vi "Main Monitor Loop.vi"(8 "error in (no error)":errorcluster, 11 "main ref":T1) -> (0 "error out":errorcluster)   [LabVIEW 2025]
uses:
  controls/LAB-IQ UI Data.ctl
panel:
  in  "millisecond multiple":u32=5
  out "Test Stop Temp":bool
  out "DepthZ":dbl
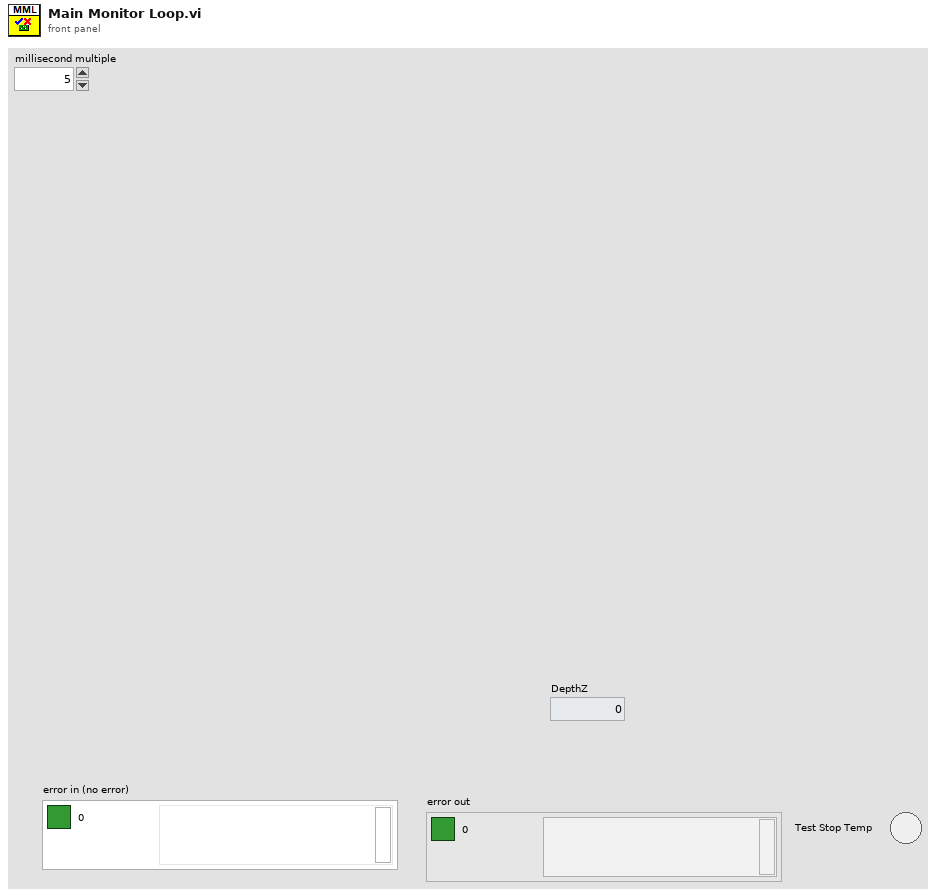
[diagram p1: front panel]
types:
  T1 = typedef "LAB-IQ UI Data.ctl" = cluster{"Main Home Screen":cluster{"GUI":refnum<vi>, "Platform Settings":refnum<vi>, "Configure":refnum<vi>, "Home":refnum<vi>, "EXIT":refnum<vi>, "service 2":refnum<vi>, "MainPage":refnum<vi>, "Analysis":refnum<vi>}, "Platform Settings":cluster{"mm/s  Surge":refnum<vi>, "Update Surge Speed":refnum<vi>, "Drive Error":refnum<vi>, "Disable Axis Jog Soft Limits":refnum<vi>, "mm/s  Sway":refnum<vi>, "Sway and Surge COM Status":refnum<vi>, "Heave COM Status":refnum<vi>, "Enable Platform":refnum<vi>, "Surge Forward Main":refnum<vi>, "Sway Right Main":refnum<vi>, "Sway Left Main":refnum<vi>, "Heave Down Main":refnum<vi>, "Heave Up main":refnum<vi>, "Update Sway Speed":refnum<vi>, "Update Heave Speed":refnum<vi>, "mm/s Heave":refnum<vi>, "mm/sec":refnum<vi>, "mm":refnum<vi>, "Surge Backward Main":refnum<vi>}, "Analysis Screen":cluster{"Analysis Home":refnum<vi>, "Surface Analysis":refnum<vi>, "Imaging":refnum<vi>, "Image Analysis":refnum<vi>, "Post Analysis":refnum<vi>}, "Config Screen":cluster{"Select Load Head":refnum<vi>, "Notes :":refnum<vi>, "FILE":refnum<vi>, "Sample ID :":refnum<vi>, "Operator ID :":refnum<vi>, "Operator Name :":refnum<vi>, "Auto":refnum<vi>}, "Motion Module":cluster{"zNL":refnum<vi>, "NL disp":refnum<vi>, "Rotary Tab":refnum<vi>, "Motion Direction:  3":refnum<vi>, "E.Velocity 2":refnum<vi>, "e.v/ssr 2":refnum<vi>, "Enter Fixed E.Velocity 2":refnum<vi>, "Enter Final SRR 2":refnum<vi>, "Enter initial SRR 2":refnum<vi>, "Enter Fixed SRR 2":refnum<vi>, "Enter the Final E.Velocity (m/s) 2":refnum<vi>, "Enter initial E.Velocity (m/s) 2":refnum<vi>, "Final Speed (RPM) 3":refnum<vi>, "Initial Speed (RPM) 2":refnum<vi>, "Enter the Final Velocity (m/s) 3":refnum<vi>, "Enter initial Velocity (m/s)  3":refnum<vi>, "Ramp Up 2":refnum<vi>, "TEST SELECTION":refnum<vi>, "SPEED SELECTION : ":refnum<vi>, "Angular Oscillation Set":refnum<vi>, "Traction":refnum<vi>, "Step Speed":refnum<vi>, "StepTable For Load-Speed":refnum<vi>, "StepTable For Speed":refnum<vi>, "Surge Forward MM":refnum<vi>, "Surge Backward MM":refnum<vi>, "M3 Image":refnum<vi>, "String 39":refnum<vi>, "Sway Left MM":refnum<vi>, "Sway Right MM":refnum<vi>, "Disable Axis Jog Soft Limits":refnum<vi>, "mm":refnum<vi>, "Heave Down MM":refnum<vi>, "Heave Up MM":refnum<vi>, "Wear Track Diameter (mm)":refnum<vi>, "Set WTD":refnum<vi>, "HomeScratch":refnum<vi>, "HomeRot":refnum<vi>, "PlaceModule":refnum<vi>, "Enter the Angle (Deg)":refnum<vi>, "Enter the Frequency (Hz)":refnum<vi>, "Motion Mode:":refnum<vi>, "LR Sway":refnum<vi>, "Rot Hor":refnum<vi>, "Scratch":refnum<vi>, "LR Cam":refnum<vi>, "MMBack":refnum<vi>, "MMNext":refnum<vi>, "Rot Ver":refnum<vi>, "Rotary Module Selection":refnum<vi>, "calculate rotary":refnum<vi>, "SPEED SELECTION : rotary":refnum<vi>, "Import 2":refnum<vi>, "Save 2":refnum<vi>, "File Path :  2":refnum<vi>, "String 45":refnum<vi>, "StepTable For Speed 3":refnum<vi>, "Enter the Speed(mm/sec)":refnum<vi>, "Enter the Speed(RPM)":refnum<vi>, "Enter Scratch Speed (mm/s):":refnum<vi>, "SwaySpeed Set":refnum<vi>, "Scartch Offset":refnum<vi>, "Motion type:":refnum<vi>, "HomeScratch 2":refnum<vi>, "Enter Scratch length (mm):":refnum<vi>, "Wear Track Diameter":refnum<vi>, "Rotary Speed Exced":refnum<vi>, "Scratch Mode":refnum<vi>, "No of Scratch":refnum<vi>}, "Environmental control":cluster{"Humidity  Status  3":refnum<vi>, "Low Temp  Status  2":refnum<vi>, "TK4 status 2":refnum<vi>, "Stage Temperature":refnum<vi>, "Sample Temperature":refnum<vi>, "Humidity (Amb)":refnum<vi>, "Clear List":refnum<vi>, "Add to list":refnum<vi>, "Wear":refnum<vi>, "Vibration":refnum<vi>, "Humidity (Chamber)":refnum<vi>, "Temperature (Chamber)":refnum<vi>, "ECR ":refnum<vi>, "Temperature (Amb)":refnum<vi>, "Microphone":refnum<vi>, "Acoustic Emission 3":refnum<vi>, "SNext":refnum<vi>, "APBack":refnum<vi>, "Enter the Temperature (°C):":refnum<vi>, "Enter the Stage \nTemperature (°C):":refnum<vi>, "Enter the Humidity (%Rh):":refnum<vi>, "Low Temp":refnum<vi>, "High Temp":refnum<vi>, "Humidity":refnum<vi>, "Sensors Picked":refnum<vi>}, "About Screen":cluster{"Password":refnum<vi>, "Home Service":refnum<vi>, "Advanced Setting":refnum<vi>, "About Tab":refnum<vi>, "ECR Port:":refnum<vi>, "Ramp Port:":refnum<vi>, "Installation/Replacement completed":refnum<vi>, "Loahead":refnum<vi>, "Heave and Surge COM Port:":refnum<vi>, "Sway COM Port:":refnum<vi>, "Temp Modbus:":refnum<vi>, "Humidity Port:":refnum<vi>, "Edit Gain Constants":refnum<vi>, "Save Gain Constants":refnum<vi>}, "Main Screen":cluster{"Main Screen Tab":refnum<vi>, "Angle and Frequency":refnum<vi>, "Stroke (mm)":refnum<vi>, "Angle (Deg)":refnum<vi>, "Main Speed Tab":refnum<vi>, "MTM MOTOR DISPLAY":refnum<vi>, "Disc Speed (m/sec)":refnum<vi>, "Ball Speed (m/sec)":refnum<vi>, "Disc Speed (RPM)":refnum<vi>, "Ball Speed (RPM)":refnum<vi>, "SPEED TAB":refnum<vi>, "Speed (m/sec)":refnum<vi>, "Set Speed (m/sec)":refnum<vi>, "Speed (RPM)":refnum<vi>, "Set Speed":refnum<vi>, "Time Tab":refnum<vi>, "Time ( HH:MM:SS ) 2":refnum<vi>, "Test Duration":refnum<vi>, "Test Duration 4":refnum<vi>, "TEST CYCLE":refnum<vi>, "TOTAL CYCLES":refnum<vi>, "Set Load (N)":refnum<vi>, "Temp Tabs":refnum<vi>, "Heater":refnum<vi>, "TK4 status":refnum<vi>, "ChamberTemp":refnum<vi>, "SetTmp":refnum<vi>, "Controller  Status":refnum<vi>, "ChamberTemp 2":refnum<vi>, "SetTmp 2":refnum<vi>, "Controller  Status 2":refnum<vi>, "ChamberTemp 3":refnum<vi>, "SetTmp 3":refnum<vi>, "Cooling":refnum<vi>, "Load Communication":refnum<vi>, "Ambient \nTemperature":refnum<vi>, "HumCOMStatus":refnum<vi>, "Ambient\n Humidity":refnum<vi>, "Freq (Hz)":refnum<vi>, "Load En":refnum<vi>, "NLt":refnum<vi>, "zNL 2":refnum<vi>, "Humidity On":refnum<vi>, "humidity disp":refnum<vi>, "Set Humidity":refnum<vi>, "NL disp 2":refnum<vi>, "Humidity On 2":refnum<vi>, "humidity disp 2":refnum<vi>, "Set Humidity 2":refnum<vi>, "NL disp 3":refnum<vi>, "AppLoadSeq scratch":refnum<vi>, "Stop Scratch":refnum<vi>, "ClrLog":refnum<vi>, "Trip Log":refnum<vi>, "STOP":refnum<vi>, "Start Test":refnum<vi>, "Test status":refnum<vi>, "AR Led":refnum<vi>, "Data":refnum<vi>, "Health":refnum<vi>, "Sway COM Status":refnum<vi>, "Heave COM Status":refnum<vi>, "Grp Tab":refnum<vi>, "Sub Graph":refnum<vi>, "SD (mm)":refnum<vi>, "Siliding distance Reset Graph":refnum<vi>, "SDGp":refnum<vi>, "Humidity Reset Graph":refnum<vi>, "HumrGp":refnum<vi>, "Acoustic Emission (mV)":refnum<vi>, "Aqucostic Reset Graph":refnum<vi>, "gACQUOS":refnum<vi>, "ECR RESET":refnum<vi>, "ECR":refnum<vi>, "Temperature Reset":refnum<vi>, "Acoustic Emission (mV) 2":refnum<vi>, "Aqucostic Reset Graph 2":refnum<vi>, "gACQUOS 2":refnum<vi>, "ECR RESET 2":refnum<vi>, "ECR 2":refnum<vi>, "Temperature Reset 2":refnum<vi>, "Temperature (deg c)":refnum<vi>, "Speed Reset Graph":refnum<vi>, "Speed Tab":refnum<vi>, "MTM DISC  SPEED":refnum<vi>, "MTM BALL SPEED":refnum<vi>, "speed mm/sec":refnum<vi>, "Hymidity":refnum<vi>, "Humidity Disable trip":refnum<vi>, "CoF Trip  2":refnum<vi>, "Depth Trip":refnum<vi>, "Weart Deapth":refnum<vi>, "Depth Reset Graph":refnum<vi>, "Weart":refnum<vi>, "Depthz":refnum<vi>, "Depth (µm)":refnum<vi>, "WearGp":refnum<vi>, "NL Trip 2":refnum<vi>, "Load pid":refnum<vi>, "Load Disable Trip":refnum<vi>, "Load Reset Graph":refnum<vi>, "NL Display 4":refnum<vi>, "Main Chart 3":refnum<vi>, "BACK":refnum<vi>, "Depth Trip 2":refnum<vi>, "COF TRIP ":refnum<vi>, "Friction Force (N)":refnum<vi>, "FF Reset Graph":refnum<vi>, "FF Disable Trip":refnum<vi>, "FF TRIP":refnum<vi>, "COF Disable Trip":refnum<vi>, "COF Reset Graph":refnum<vi>, "Start Test Temp":refnum<vi>, "zFF":refnum<vi>, "Friction Force (N) Graph":refnum<vi>, "Coefficient of Friction":refnum<vi>, "Scratch Start Test":refnum<vi>, "FF Tab":refnum<vi>, "Cyclic Friction Force (N)":refnum<vi>, "CZ FF":refnum<vi>, "Cyclic Friction Force (N) Graph":refnum<vi>, "Cyclic Coefficient of Friction":refnum<vi>, "Cyclic FF TRIP":refnum<vi>, "Cyclic FF Disable Trip":refnum<vi>, "cyclic COF Disable Trip":refnum<vi>, "cyclic COF TRIP":refnum<vi>, "cyclic COF Reset Graph":refnum<vi>, "Cyclic FF Reset Graph":refnum<vi>, "Test Trip":refnum<vi>, "Multi Scratch Pass":refnum<vi>}, "Loading":cluster{"Indentation":refnum<vi>, "Reference Sample":refnum<vi>, "Load Cell Communication Slide":refnum<vi>, "com 3":refnum<vi>, "com":refnum<vi>, "DecaForce COM Status":refnum<vi>, "Update":refnum<vi>, "Clear 3":refnum<vi>, "seq":refnum<vi>, "Stribeck table":refnum<vi>, "Stribeck Table  For loading":refnum<vi>, "Loading Mode":refnum<vi>, "Enter the Final Load (N)":refnum<vi>, "Enter the CoF Trip":refnum<vi>, "Enter the Friction Force Trip":refnum<vi>, "Enter the Normal load Trip":refnum<vi>, "Enter the Load  (N)":refnum<vi>, "KiloForce":refnum<vi>, "DecaForce ":refnum<vi>, "MicroForce":refnum<vi>, "LHBack":refnum<vi>, "LHNext":refnum<vi>, "Enter the Loading Rate (N/min)":refnum<vi>, "Message":refnum<vi>, "Warning 2":refnum<vi>, "SSP 0.75":refnum<vi>, "SSP 0.5":refnum<vi>, "SSP 0.3":refnum<vi>, "Warning":refnum<vi>, "gui GIF":refnum<vi>, "Communication is established":refnum<vi>, "AppLoad 4":refnum<vi>, "Multipoint":refnum<vi>, "Load Selection":refnum<vi>}, "PID":cluster{"Ramp MulFac":refnum<vi>, "pulses LoadDiffRamp(2..10)":refnum<vi>, "PulseControlRamp(diff<=3N)":refnum<vi>, "SetLoadDeadband(%) Load(0-10N)":refnum<vi>, "PID gains out delay (microForce)":refnum<vi>, "Ramp":refnum<vi>, "Gain 2":refnum<vi>, "pulses LoadDiff(2..10)":refnum<vi>, "pulses LoadDiff(11..50)":refnum<vi>, "PulseControl(diff<=3N)":refnum<vi>, "SetLoadDeadband(%)  2":refnum<vi>, "Dummy Run":refnum<vi>, "Vertical load (N)":refnum<vi>, "AutoTune":refnum<vi>, "Offset 3 ":refnum<vi>, "apply load":refnum<vi>, "Offset  3":refnum<vi>, "apply load 2":refnum<vi>, "Enter ByPass Load":refnum<vi>, "reinit 3":refnum<vi>, "output range delay":refnum<vi>, "PID gains out delay":refnum<vi>, "Bypass Load":refnum<vi>, "pulsesSent":refnum<vi>, "pulses ":refnum<vi>, "actpid":refnum<vi>, "gFF Rot":refnum<vi>, "pulses LoadDiff(21..1000)":refnum<vi>, "Delay":refnum<vi>, "deadband":refnum<vi>}, "Config Parameters":cluster{"Tab Control 3":refnum<vi>, "Tab Control 19":refnum<vi>, "SAMPLES":refnum<vi>, "Re-initilaize":refnum<vi>, "Filter ON/OFF":refnum<vi>, "TracHomeSurgeOffsetCounts 10MM":refnum<vi>, "TracHomeSwayOffsetCounts 10MM":refnum<vi>, "Acoustic Emission:":refnum<vi>, "Apply Filter (FF)":refnum<vi>, "Filter% 2":refnum<vi>, "Apply Filter (Load)":refnum<vi>, "Filter% ":refnum<vi>, "Sway distance (mm)":refnum<vi>, "Surge distance (mm)":refnum<vi>, "DataSavingLoopDelay(ms)":refnum<vi>, "SAVE 2":refnum<vi>, "Enter Distance":refnum<vi>, "Sway Counts:":refnum<vi>, "Distance (mm): 3":refnum<vi>, "Surge Counts:":refnum<vi>, "Distance (mm): 2":refnum<vi>, "Distance (mm):":refnum<vi>, "Heave Counts:":refnum<vi>, "LRMHomeSurgeOffsetCounts":refnum<vi>, "LRMHomeSwayOffsetCounts":refnum<vi>, "TracHomeSurgeOffsetCounts 20MM":refnum<vi>, "TracHomeSwayOffsetCounts 20MM":refnum<vi>, "RotHomeSwayOffsetCounts":refnum<vi>, "RotHomeSurgeOffsetCounts":refnum<vi>, "Heave distance":refnum<vi>, "Zmm":refnum<vi>, "Heave Pulses/mm":refnum<vi>, "Surge Pulses/mm":refnum<vi>, "Sway Pulses/mm":refnum<vi>, "Heave Pitch":refnum<vi>, "Surge Pitch":refnum<vi>, "Sway Pitch":refnum<vi>, "Heave PPR":refnum<vi>, "Surge PPR":refnum<vi>, "Sway PPR":refnum<vi>, "Tab Control 5":refnum<vi>, "Tab Control 14":refnum<vi>, "Tab Control 26":refnum<vi>, "AE":refnum<vi>, "Heave Loop Delay":refnum<vi>, "Heave PID Speed":refnum<vi>, "Surge Jog Speed":refnum<vi>, "Heave Jog Speed":refnum<vi>, "Sway Loop Delay":refnum<vi>, "Sway PID Speed":refnum<vi>, "Sway Jog Speed":refnum<vi>}, "Loading Com Port":cluster{"ClearAll":refnum<vi>, "Mz(Nm)":refnum<vi>, "My(Nm)":refnum<vi>, "Mx(Nm)":refnum<vi>, "Save Dwell":refnum<vi>, "Mx ":refnum<vi>, "My ":refnum<vi>, "Mz":refnum<vi>, "Fx(N)":refnum<vi>, "Fy(N)":refnum<vi>, "Fz(N)":refnum<vi>, "ZeroAll":refnum<vi>, "Acq Delay (ms)":refnum<vi>, "Burst Delay (ms)":refnum<vi>, "model":refnum<vi>, "SN":refnum<vi>, "FFx(N)":refnum<vi>, "Sensor IP":refnum<vi>, "Port":refnum<vi>, "FFy(N)":refnum<vi>, "Load(N)":refnum<vi>, "delete Handle":refnum<vi>, "Create Handle":refnum<vi>, "ft_data":refnum<vi>, "ft_range":refnum<vi>, "ft_data 2":refnum<vi>, "stop 6":refnum<vi>, "running_flag":refnum<vi>, "ft_udp_handle":refnum<vi>, "get-data-return":refnum<vi>, "get-range-return":refnum<vi>, "zero-return":refnum<vi>, "filter-return":refnum<vi>, "initial-return":refnum<vi>, "deleteHandle-result":refnum<vi>, "Load Cell Temp":refnum<vi>}, "Heave AND Surge":cluster{"SURGE POSE":refnum<vi>, "error out Read":refnum<vi>, "HEAVE POSE":refnum<vi>, "State":refnum<vi>, "Homed":refnum<vi>, "Sequence ID":refnum<vi>, "error out Write":refnum<vi>, "faultCode":refnum<vi>, "Ack ID":refnum<vi>, "SPEED":refnum<vi>, "Distance":refnum<vi>, "Mode Command":refnum<vi>, "Heave and Surge Read":refnum<vi>, "Read Heave Temp":refnum<vi>, "Spare 15":refnum<vi>, "Spare 14":refnum<vi>, "Spare 13":refnum<vi>, "Spare 12":refnum<vi>, "Spare 11":refnum<vi>, "Spare 10":refnum<vi>, "Spare 9":refnum<vi>, "Spare 8":refnum<vi>, "Spare 7":refnum<vi>, "Spare 6":refnum<vi>, "Spare 5":refnum<vi>, "Spare 4":refnum<vi>, "Spare 2":refnum<vi>, "Spare 1":refnum<vi>, "Node Id":refnum<vi>, "Spare 3":refnum<vi>, "SPARE 4":refnum<vi>, "SPARE 3":refnum<vi>, "SPARE 2":refnum<vi>, "SPARE 1":refnum<vi>, "fwMajor":refnum<vi>, "fwMinor":refnum<vi>, "Manual Write":refnum<vi>, "Heave and Surge Write":refnum<vi>}, "New PID LOGIC":cluster{"Fine Tune Zone":refnum<vi>, "PID SDelay":refnum<vi>, "Max_pos_limit":refnum<vi>, "Min_pos_limit":refnum<vi>, "i_limit":refnum<vi>, "pct_scale":refnum<vi>, "Deadband":refnum<vi>, "Kd":refnum<vi>, "Ki":refnum<vi>, "Kp":refnum<vi>, "Current Position":refnum<vi>, "Set Load":refnum<vi>, "Current Load":refnum<vi>, "Pulse delta":refnum<vi>, "Init Step":refnum<vi>, "Max Step Linit":refnum<vi>}, "SWAY ":cluster{"fwMajor":refnum<vi>, "Homed":refnum<vi>, "Rotary POSE":refnum<vi>, "State":refnum<vi>, "SWAY POSE":refnum<vi>, "Ack ID":refnum<vi>, "faultCode":refnum<vi>, "Node Id":refnum<vi>, "fwMinor":refnum<vi>, "Spare 6":refnum<vi>, "Spare 5":refnum<vi>, "Spare 4":refnum<vi>, "Spare 3":refnum<vi>, "Spare 2":refnum<vi>, "Spare 1":refnum<vi>, "Spare 7":refnum<vi>, "SPARE  5":refnum<vi>, "error out Write  SWAY ":refnum<vi>, "error out Read SWAY ":refnum<vi>, "Manual Write SWAY ":refnum<vi>, "SWAY WRITE":refnum<vi>, "SPARE  4":refnum<vi>, "SPARE  3":refnum<vi>, "SPARE 2":refnum<vi>, "SPARE 1":refnum<vi>, "Spare 15":refnum<vi>, "Spare 14":refnum<vi>, "Spare 13":refnum<vi>, "Spare 12":refnum<vi>, "Spare 11":refnum<vi>, "Spare 9":refnum<vi>, "Spare 8":refnum<vi>, "SPEED":refnum<vi>, "Distance":refnum<vi>, "Mode Command":refnum<vi>, "Sequence ID":refnum<vi>, "SWAY READ":refnum<vi>, "Spare 10":refnum<vi>, "Read SWAY Temp":refnum<vi>}, "Analysis Screen":cluster{"Analysis Home":refnum<vi>, "Refresh 2":refnum<vi>, "MEAN 4":refnum<vi>, "SD 4":refnum<vi>, "VARIANCE 4":refnum<vi>, "MEAN  3":refnum<vi>, "SD  3":refnum<vi>, "VARIANCE  3":refnum<vi>, "MEAN 2":refnum<vi>, "SD  2":refnum<vi>, "VARIANCE 2":refnum<vi>, "MEAN":refnum<vi>, "SD":refnum<vi>, "VARIANCE":refnum<vi>, "File 4 Discription":refnum<vi>, "OPEN 4":refnum<vi>, "File Name 4":refnum<vi>, "OPEN 3":refnum<vi>, "File 3 Discription":refnum<vi>, "File Name 3":refnum<vi>, "Y-AXIS":refnum<vi>, "X-AXIS":refnum<vi>, "XY Graph":refnum<vi>, "File Name 2":refnum<vi>, "File Name 1":refnum<vi>, "OPEN 2":refnum<vi>, "OPEN 1":refnum<vi>, "File 1 Discription ":refnum<vi>, "File 2 Discription":refnum<vi>}}
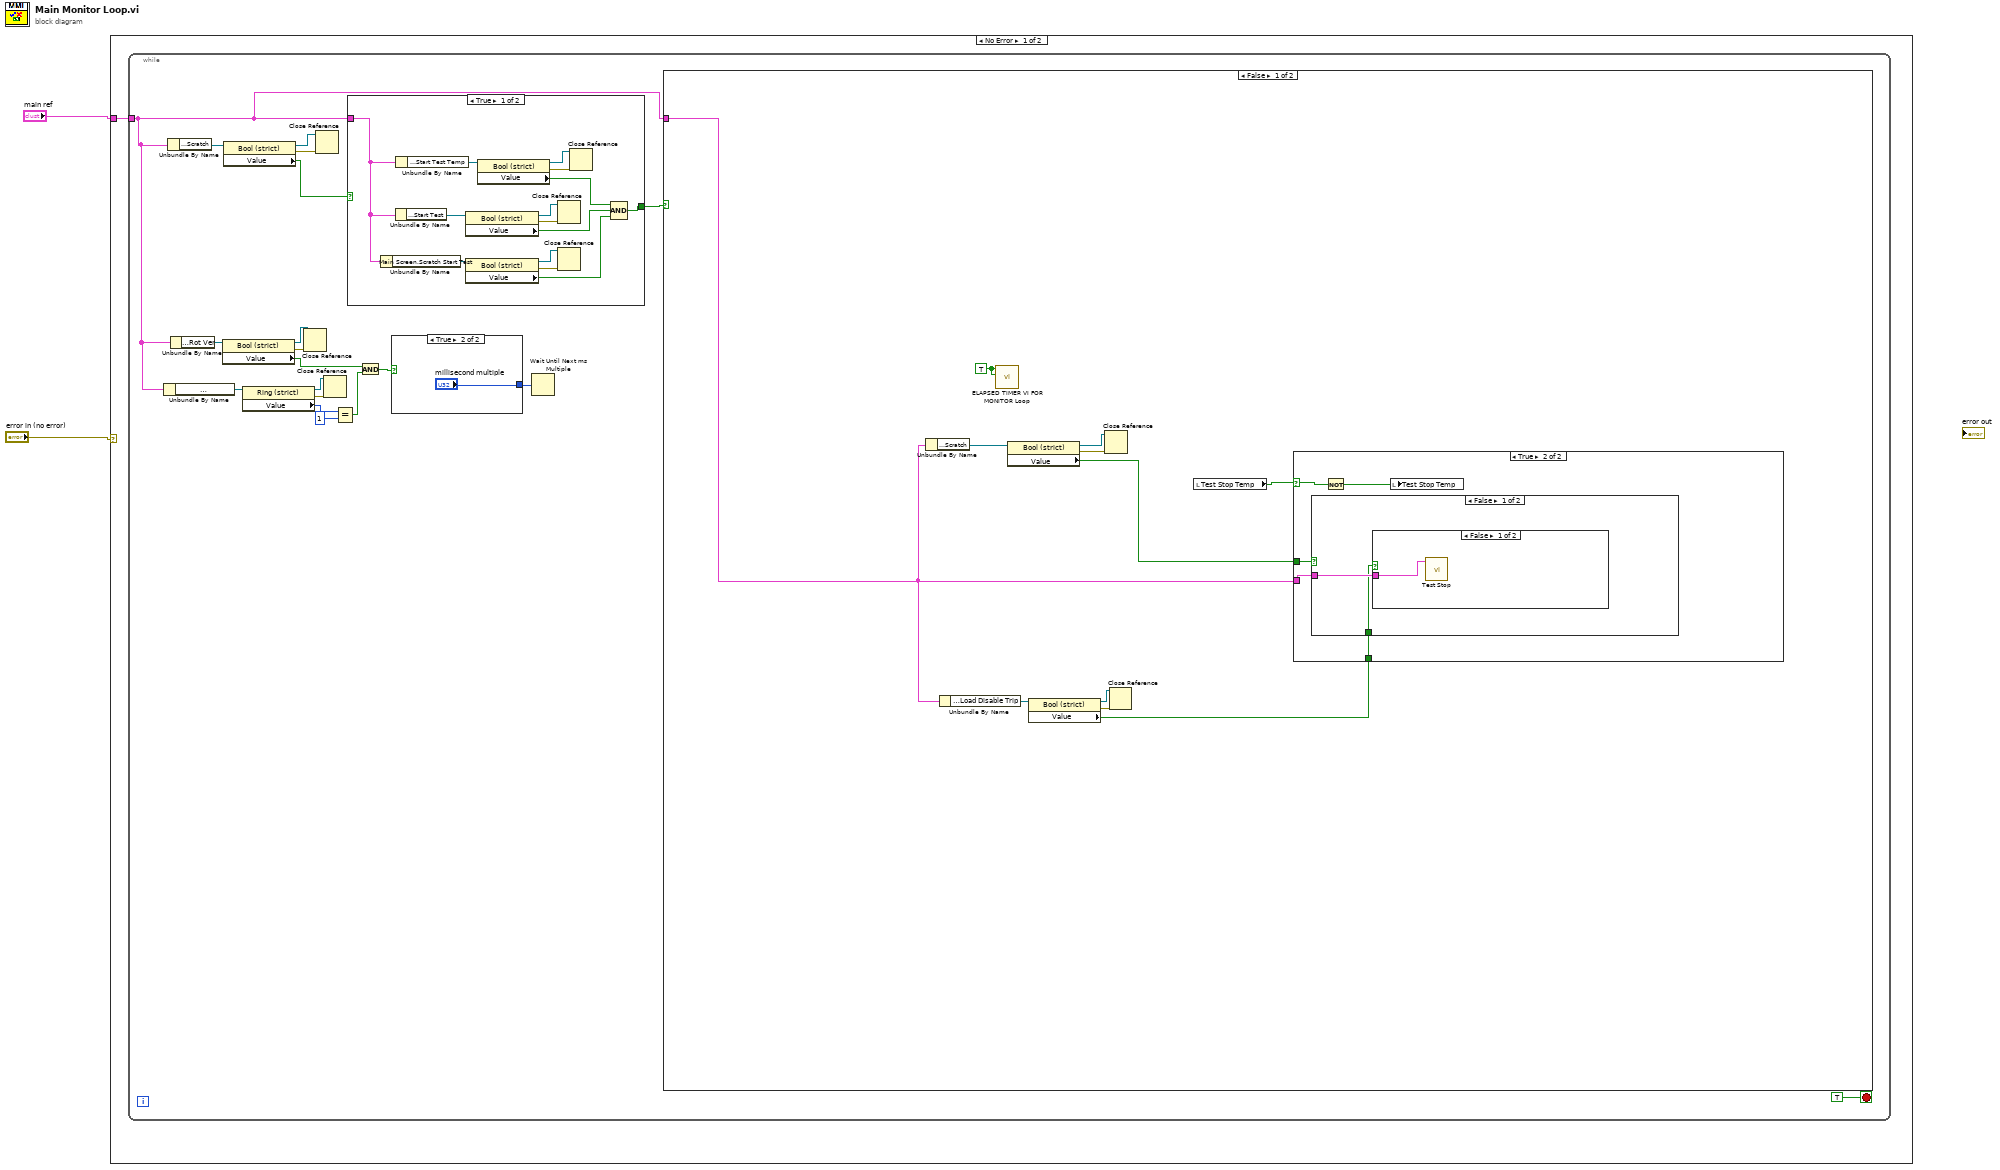
[diagram p0: block diagram]
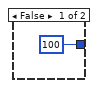
[diagram p2: hidden frame]
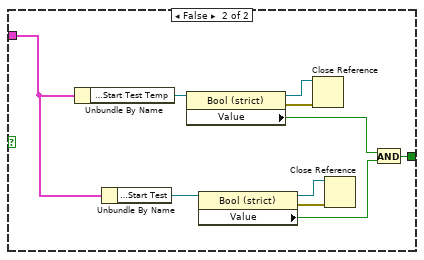
[diagram p3: hidden frame]
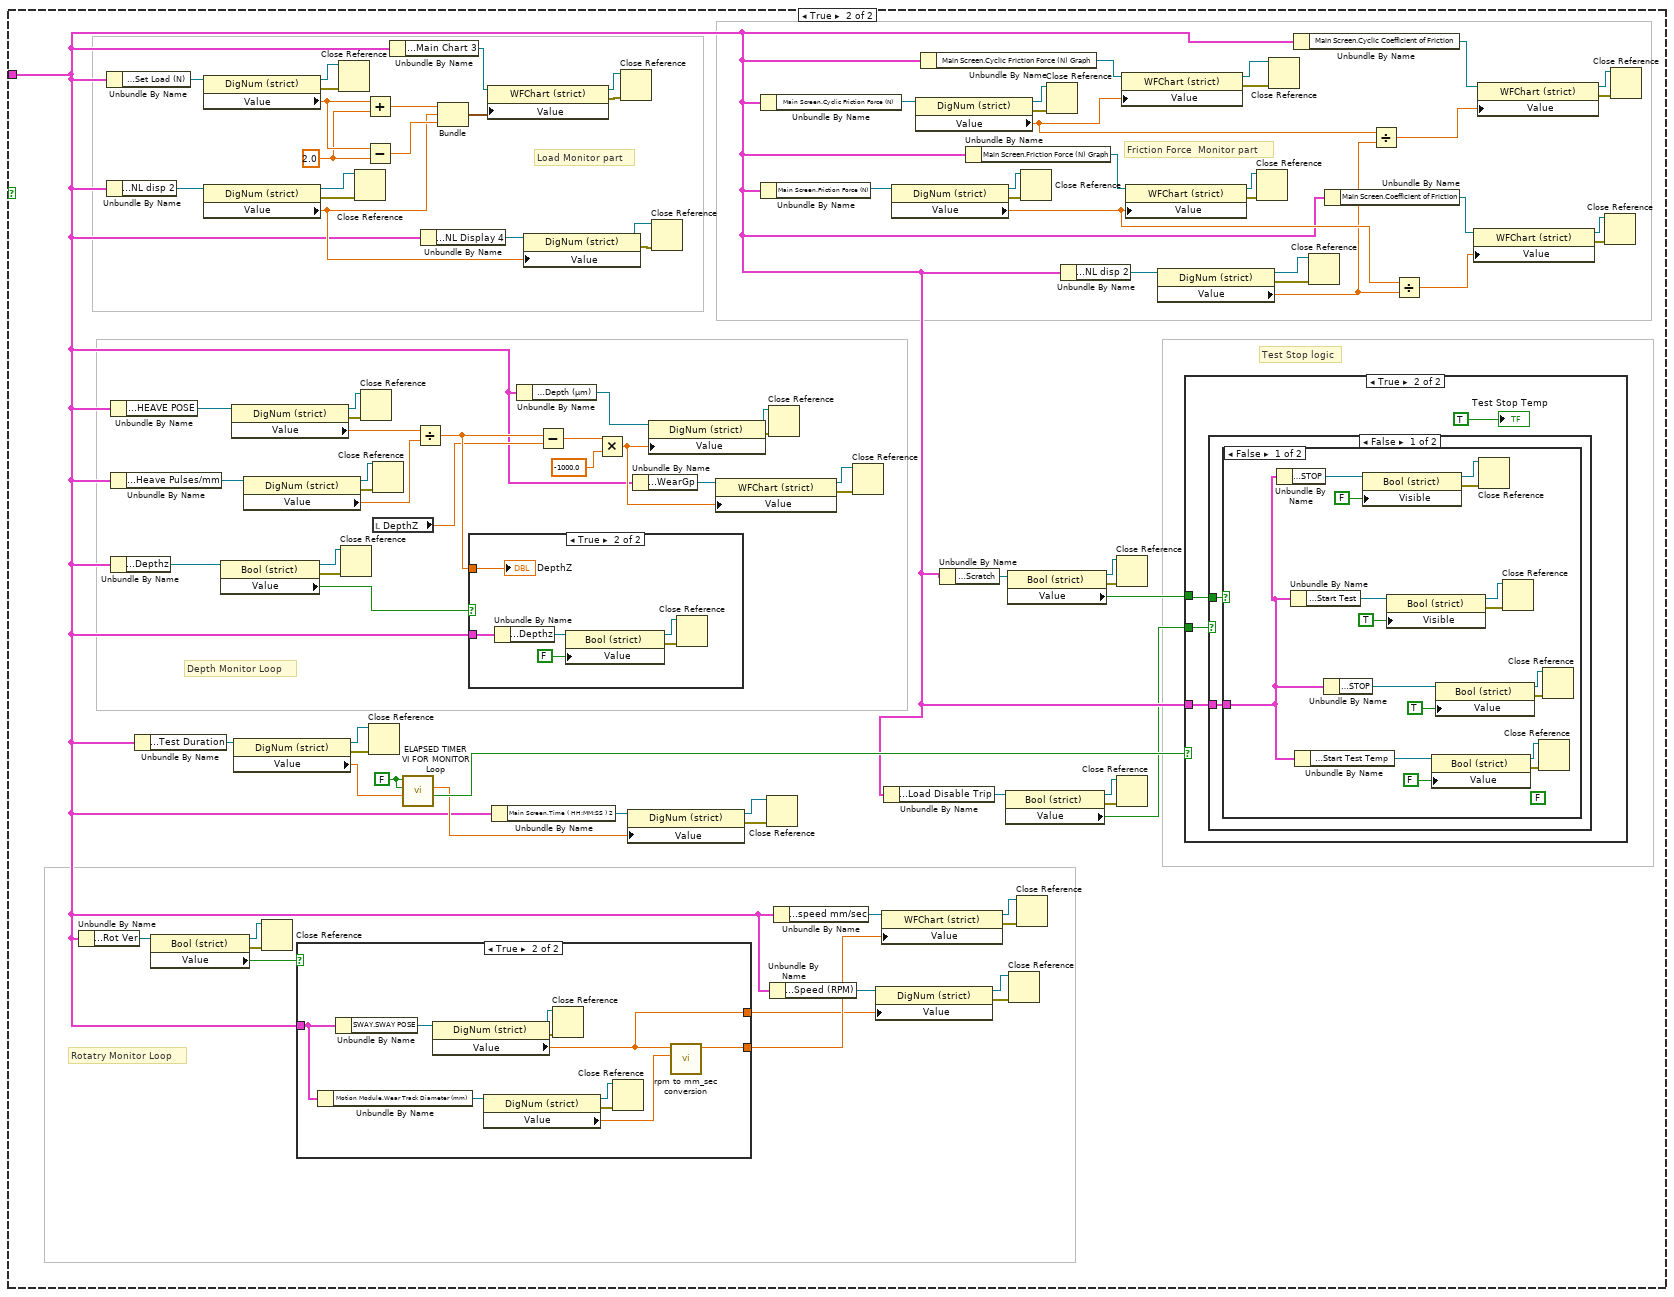
[diagram p7: hidden frame]
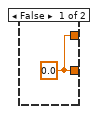
[diagram p8: hidden frame]
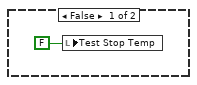
[diagram p9: hidden frame]
diagram:
  n1 = case shown="No Error" "error in (no error)" {
    tunnel: "main ref" -> [w3 _]
    frame No Error {
      n2 = while {
        tunnel: w3 -> [w5]
        stop <- TRUE stop-if-true
        n3 = Unbundle By Name(w5) -> ("Motion Module.Motion Mode:"=w10:refnum<vi>)
        n4 = Unbundle By Name(w5) -> ("Motion Module.Scratch"=w19:refnum<vi>)
        n5 = Unbundle By Name(w5) -> ("Motion Module.Rot Ver"=w15:refnum<vi>)
        n6 = property class="Bool (strict)"(reference=w15) -> (reference out=w13:refnum<vi>, error out=w14:errorcluster, "Value"=w7:bool)  [unwired: 1 in]
        n7 = property class="Bool (strict)"(reference=w19) -> (reference out=w20:refnum<vi>, error out=w18:errorcluster, "Value"=w17:bool)  [unwired: 1 in]
        n8 = property class="Ring (strict)"(reference=w10) -> (reference out=w12:refnum<vi>, error out=w11:errorcluster, "Value"=w9:u16)  [unwired: 1 in]
        n9 = Close Reference(reference=w13, error in (no error)=w14) -> ()  [unwired: 1 out]
        n10 = Close Reference(reference=w20, error in (no error)=w18) -> ()  [unwired: 1 out]
        n11 = Close Reference(reference=w12, error in (no error)=w11) -> ()  [unwired: 1 out]
        n12 = Equal?(x=w9, y=u16 1) -> (x = y?=w6:bool)
        n13 = case shown="True" w17 {
          tunnel: w5 -> [w26 w42]
          tunnel: [w30 w40] -> w21
          frame True {
            n14 = Unbundle By Name(w26) -> ("Main Screen.Scratch Start Test"=w28:refnum<vi>)
            n15 = Unbundle By Name(w26) -> ("Main Screen.Start Test"=w34:refnum<vi>)
            n16 = Unbundle By Name(w26) -> ("Main Screen.Start Test Temp"=w37:refnum<vi>)
            n17 = property class="Bool (strict)"(reference=w34) -> (reference out=w33:refnum<vi>, error out=w35:errorcluster, "Value"=w31:bool)  [unwired: 1 in]
            n18 = property class="Bool (strict)"(reference=w28) -> (reference out=w29:refnum<vi>, error out=w27:errorcluster, "Value"=w25:bool)  [unwired: 1 in]
            n19 = property class="Bool (strict)"(reference=w37) -> (reference out=w38:refnum<vi>, error out=w36:errorcluster, "Value"=w32:bool)  [unwired: 1 in]
            n20 = Close Reference(reference=w33, error in (no error)=w35) -> ()  [unwired: 1 out]
            n21 = Close Reference(reference=w29, error in (no error)=w27) -> ()  [unwired: 1 out]
            n22 = Close Reference(reference=w38, error in (no error)=w36) -> ()  [unwired: 1 out]
            n23 = Compound Arithmetic op=AND(w32, w31, w25) -> (w30:bool)
          }
          frame False {
            n24 = Unbundle By Name(w42) -> ("Main Screen.Start Test Temp"=w47:refnum<vi>)
            n25 = Unbundle By Name(w42) -> ("Main Screen.Start Test"=w44:refnum<vi>)
            n26 = property class="Bool (strict)"(reference=w47) -> (reference out=w48:refnum<vi>, error out=w46:errorcluster, "Value"=w41:bool)  [unwired: 1 in]
            n27 = property class="Bool (strict)"(reference=w44) -> (reference out=w43:refnum<vi>, error out=w45:errorcluster, "Value"=w39:bool)  [unwired: 1 in]
            n28 = Close Reference(reference=w48, error in (no error)=w46) -> ()  [unwired: 1 out]
            n29 = Close Reference(reference=w43, error in (no error)=w45) -> ()  [unwired: 1 out]
            n30 = And(x=w41, y=w39) -> (x .and. y?=w40:bool)
          }
        }
        n31 = And(x=w7, y=w6) -> (x .and. y?=w4:bool)
        n32 = case shown="True" w4 {
          tunnel: [u32 100 ("millisecond multiple") "millisecond multiple"] -> w16
          frame False {
          }
          frame True {
          }
        }
        n33 = Wait Until Next ms Multiple(millisecond multiple=w16) -> ()  [unwired: 1 out]
        n34 = case shown="False" w21 {
          tunnel: w5 -> [w50 w69]
          frame False {
            w59 = TRUE ("PAUSE")
            n35 = Unbundle By Name(w50) -> ("Motion Module.Scratch"=w57:refnum<vi>)
            n36 = Unbundle By Name(w50) -> ("Main Screen.Load Disable Trip"=w51:refnum<vi>)
            n37 = call "ELAPSED TIMER VI FOR MONITOR Loop.vi"("RESET"=w59, "PAUSE"=w59) -> ()  [unwired: 7 in, 3 out]
            n38 = property class="Bool (strict)"(reference=w57) -> (reference out=w55:refnum<vi>, error out=w56:errorcluster, "Value"=w54:bool)  [unwired: 1 in]
            n39 = property class="Bool (strict)"(reference=w51) -> (reference out=w53:refnum<vi>, error out=w52:errorcluster, "Value"=w49:bool)  [unwired: 1 in]
            n40 = Close Reference(reference=w55, error in (no error)=w56) -> ()  [unwired: 1 out]
            n41 = Close Reference(reference=w53, error in (no error)=w52) -> ()  [unwired: 1 out]
            n42 = local read "Test Stop Temp"() -> (w58:bool)
            n43 = case shown="True" w58 {
              selector: w58 -> [_ w64]
              tunnel: w50 -> [_ w62]
              tunnel: w54 -> [_ w61]
              tunnel: w49 -> [_ w60]
              frame False {
              }
              frame True {
                n44 = case shown="False" w61 {
                  tunnel: w62 -> [w66 _]
                  tunnel: w60 -> [w65 _]
                  frame False {
                    n45 = case shown="False" w65 {
                      tunnel: w66 -> [w67 _]
                      frame False {
                        n46 = call "Test Stop.vi"("Data Cluster"=w67) -> ()  [unwired: 10 in, 1 out]
                      }
                      frame True {
                      }
                    }
                  }
                  frame True {
                  }
                }
                n47 = Not(x=w64) -> (.not. x?=w63:bool)
                n48 = local write "Test Stop Temp"(w63) -> ()
              }
            }
          }
          frame True {
            w125 = FALSE ("PAUSE")
            w153 = 2.0 ("y")
            # "Rotatry Monitor Loop"
            # "Test Stop logic"
            # "Depth Monitor Loop"
            # "Friction Force  Monitor part"
            # "Load Monitor part"
            n49 = Unbundle By Name(w69) -> ("Motion Module.Rot Ver"=w84:refnum<vi>)
            n50 = Unbundle By Name(w69) -> ("Main Screen.Set Load (N)"=w155:refnum<vi>)
            n51 = Unbundle By Name(w69) -> ("Main Screen.NL disp 2"=w165:refnum<vi>)
            n52 = Unbundle By Name(w69) -> ("Heave AND Surge.HEAVE POSE"=w147:refnum<vi>)
            n53 = Unbundle By Name(w69) -> ("Config Parameters.Heave Pulses/mm"=w144:refnum<vi>)
            n54 = Unbundle By Name(w69) -> ("Main Screen.Depthz"=w139:refnum<vi>)
            n55 = Unbundle By Name(w69) -> ("Main Screen.Test Duration"=w123:refnum<vi>)
            n56 = property class="Bool (strict)"(reference=w84) -> (reference out=w82:refnum<vi>, error out=w83:errorcluster, "Value"=w81:bool)  [unwired: 1 in]
            n57 = property class="DigNum (strict)"(reference=w155) -> (reference out=w149:refnum<vi>, error out=w156:errorcluster, "Value"=w154:dbl)  [unwired: 1 in]
            n58 = property class="DigNum (strict)"(reference=w165) -> (reference out=w163:refnum<vi>, error out=w164:errorcluster, "Value"=w100:dbl)  [unwired: 1 in]
            n59 = property class="Bool (strict)"(reference=w139) -> (reference out=w140:refnum<vi>, error out=w138:errorcluster, "Value"=w137:bool)  [unwired: 1 in]
            n60 = property class="DigNum (strict)"(reference=w147) -> (reference out=w148:refnum<vi>, error out=w146:errorcluster, "Value"=w142:sgl)  [unwired: 1 in]
            n61 = property class="DigNum (strict)"(reference=w123) -> (reference out=w124:refnum<vi>, error out=w122:errorcluster, "Value"=w121:dbl)  [unwired: 1 in]
            n62 = property class="DigNum (strict)"(reference=w144) -> (reference out=w143:refnum<vi>, error out=w145:errorcluster, "Value"=w141:dbl)  [unwired: 1 in]
            n63 = Close Reference(reference=w82, error in (no error)=w83) -> ()  [unwired: 1 out]
            n64 = case shown="True" w81 {
              tunnel: w69 -> [_ w170]
              tunnel: [w166 w168] -> w77
              tunnel: [w166 w167] -> w73
              frame False {
                w166 = 0.0 ("Enter initial Velocity (m/s)  4")
              }
              frame True {
                n65 = Unbundle By Name(w170) -> ("Motion Module.Wear Track Diameter (mm)"=w173:refnum<vi>)
                n66 = Unbundle By Name(w170) -> ("SWAY.SWAY POSE"=w174:refnum<vi>)
                n67 = property class="DigNum (strict)"(reference=w174) -> (reference out=w176:refnum<vi>, error out=w175:errorcluster, "Value"=w167:sgl)  [unwired: 1 in]
                n68 = property class="DigNum (strict)"(reference=w173) -> (reference out=w171:refnum<vi>, error out=w172:errorcluster, "Value"=w169:dbl)  [unwired: 1 in]
                n69 = Close Reference(reference=w176, error in (no error)=w175) -> ()  [unwired: 1 out]
                n70 = Close Reference(reference=w171, error in (no error)=w172) -> ()  [unwired: 1 out]
                n71 = call "rpm to mm_sec conversion.vi"("Wear Track Diameter"=w169, "Initial Speed (RPM)"=w167) -> ("Enter initial Velocity (m/s)  4"=w168:dbl)  [unwired: 7 in, 2 out]
              }
            }
            n72 = Close Reference(reference=w149, error in (no error)=w156) -> ()  [unwired: 1 out]
            n73 = Close Reference(reference=w140, error in (no error)=w138) -> ()  [unwired: 1 out]
            n74 = Close Reference(reference=w163, error in (no error)=w164) -> ()  [unwired: 1 out]
            n75 = Close Reference(reference=w148, error in (no error)=w146) -> ()  [unwired: 1 out]
            n76 = Add(x=w154, y=w153) -> (x+y=w152:dbl)
            n77 = Subtract(x=w154, y=w153) -> (x-y=w151:dbl)
            n78 = Close Reference(reference=w124, error in (no error)=w122) -> ()  [unwired: 1 out]
            n79 = Close Reference(reference=w143, error in (no error)=w145) -> ()  [unwired: 1 out]
            n80 = local read "DepthZ"() -> (w135:dbl)
            n81 = Unbundle By Name(w69) -> ("Main Screen.Main Chart 3"=w159:refnum<vi>)
            n82 = call "ELAPSED TIMER VI FOR MONITOR Loop.vi"("TARGET"=w121, "RESET"=w125, "PAUSE"=w125) -> ("ELAPSED INDICATION"=w108:bool, "ELAPSED TIMER"=w86:dbl)  [unwired: 6 in, 1 out]
            n83 = Divide(x=w142, y=w141) -> (x/y=w136:dbl)
            n84 = Unbundle By Name(w69) -> ("Main Screen.NL Display 4"=w160:refnum<vi>)
            n85 = Bundle(w152, "Value"=w100, w151) -> (w150:cluster{dbl, "Value":dbl, dbl})  [unwired: 1 in]
            n86 = case shown="True" w137 {
              tunnel: w136 -> [_ w206]
              tunnel: w69 -> [_ w202]
              frame False {
              }
              frame True {
                n87 = Unbundle By Name(w202) -> ("Main Screen.Depthz"=w204:refnum<vi>)
                n88 = property class="Bool (strict)"(reference=w204, "Value"=FALSE) -> (reference out=w203:refnum<vi>, error out=w205:errorcluster)  [unwired: 1 in]
                n89 = Close Reference(reference=w203, error in (no error)=w205) -> ()  [unwired: 1 out]
                "DepthZ" <- w206
              }
            }
            n90 = property class="WFChart (strict)"(reference=w159, "Value"=w150) -> (reference out=w157:refnum<vi>, error out=w158:errorcluster)  [unwired: 1 in]
            n91 = Unbundle By Name(w69) -> ("Main Screen.Time ( HH:MM:SS ) 2"=w87:refnum<vi>)
            n92 = Unbundle By Name(w69) -> ("Main Screen.Depth (µm)"=w133:refnum<vi>)
            n93 = property class="DigNum (strict)"(reference=w160, "Value"=w100) -> (reference out=w162:refnum<vi>, error out=w161:errorcluster)  [unwired: 1 in]
            n94 = Subtract(x=w136, y=w135) -> (x-y=w127:dbl)
            n95 = Multiply(x=w127, y=-1000.0) -> (x*y=w128:dbl)
            n96 = Close Reference(reference=w157, error in (no error)=w158) -> ()  [unwired: 1 out]
            n97 = property class="DigNum (strict)"(reference=w87, "Value"=w86) -> (reference out=w119:refnum<vi>, error out=w120:errorcluster)  [unwired: 1 in]
            n98 = Unbundle By Name(w69) -> ("Main Screen.WearGp"=w130:refnum<vi>)
            n99 = property class="DigNum (strict)"(reference=w133, "Value"=w128) -> (reference out=w134:refnum<vi>, error out=w132:errorcluster)  [unwired: 1 in]
            n100 = Close Reference(reference=w162, error in (no error)=w161) -> ()  [unwired: 1 out]
            n101 = property class="WFChart (strict)"(reference=w130, "Value"=w128) -> (reference out=w131:refnum<vi>, error out=w129:errorcluster)  [unwired: 1 in]
            n102 = Unbundle By Name(w69) -> ("Main Screen.Cyclic Friction Force (N)"=w104:refnum<vi>)
            n103 = Unbundle By Name(w69) -> ("Main Screen.Friction Force (N)"=w117:refnum<vi>)
            n104 = Close Reference(reference=w119, error in (no error)=w120) -> ()  [unwired: 1 out]
            n105 = Close Reference(reference=w134, error in (no error)=w132) -> ()  [unwired: 1 out]
            n106 = Unbundle By Name(w69) -> ("Main Screen.Speed (RPM)"=w76:refnum<vi>)
            n107 = Unbundle By Name(w69) -> ("Main Screen.speed mm/sec"=w78:refnum<vi>)
            n108 = Close Reference(reference=w131, error in (no error)=w129) -> ()  [unwired: 1 out]
            n109 = property class="DigNum (strict)"(reference=w76, "Value"=w73) -> (reference out=w74:refnum<vi>, error out=w75:errorcluster)  [unwired: 1 in]
            n110 = property class="WFChart (strict)"(reference=w78, "Value"=w77) -> (reference out=w80:refnum<vi>, error out=w79:errorcluster)  [unwired: 1 in]
            n111 = Unbundle By Name(w69) -> ("Main Screen.Load Disable Trip"=w70:refnum<vi>)
            n112 = property class="DigNum (strict)"(reference=w117) -> (reference out=w118:refnum<vi>, error out=w116:errorcluster, "Value"=w110:dbl)  [unwired: 1 in]
            n113 = property class="DigNum (strict)"(reference=w104) -> (reference out=w102:refnum<vi>, error out=w103:errorcluster, "Value"=w101:dbl)  [unwired: 1 in]
            n114 = Unbundle By Name(w69) -> ("Main Screen.Cyclic Friction Force (N) Graph"=w107:refnum<vi>)
            n115 = Unbundle By Name(w69) -> ("Motion Module.Scratch"=w85:refnum<vi>)
            n116 = Unbundle By Name(w69) -> ("Main Screen.Friction Force (N) Graph"=w88:refnum<vi>)
            n117 = property class="Bool (strict)"(reference=w70) -> (reference out=w72:refnum<vi>, error out=w71:errorcluster, "Value"=w68:bool)  [unwired: 1 in]
            n118 = property class="Bool (strict)"(reference=w85) -> (reference out=w94:refnum<vi>, error out=w95:errorcluster, "Value"=w93:bool)  [unwired: 1 in]
            n119 = Close Reference(reference=w74, error in (no error)=w75) -> ()  [unwired: 1 out]
            n120 = Close Reference(reference=w80, error in (no error)=w79) -> ()  [unwired: 1 out]
            n121 = Close Reference(reference=w118, error in (no error)=w116) -> ()  [unwired: 1 out]
            n122 = Close Reference(reference=w102, error in (no error)=w103) -> ()  [unwired: 1 out]
            n123 = Unbundle By Name(w69) -> ("Main Screen.NL disp 2"=w92:refnum<vi>)
            n124 = Close Reference(reference=w94, error in (no error)=w95) -> ()  [unwired: 1 out]
            n125 = Close Reference(reference=w72, error in (no error)=w71) -> ()  [unwired: 1 out]
            n126 = property class="WFChart (strict)"(reference=w107, "Value"=w101) -> (reference out=w105:refnum<vi>, error out=w106:errorcluster)  [unwired: 1 in]
            n127 = property class="WFChart (strict)"(reference=w88, "Value"=w110) -> (reference out=w114:refnum<vi>, error out=w115:errorcluster)  [unwired: 1 in]
            n128 = property class="DigNum (strict)"(reference=w92) -> (reference out=w90:refnum<vi>, error out=w91:errorcluster, "Value"=w89:dbl)  [unwired: 1 in]
            n129 = case shown="True" w108 {
              tunnel: w69 -> [_ w180]
              tunnel: w93 -> [_ w179]
              tunnel: w68 -> [_ w178]
              frame False {
                n130 = local write "Test Stop Temp"(FALSE ("Test Stop Temp")) -> ()
              }
              frame True {
                n131 = case shown="False" w178 {
                  tunnel: w180 -> [w183 _]
                  tunnel: w179 -> [w182 _]
                  frame False {
                    n132 = case shown="False" w182 {
                      tunnel: w183 -> [w184 _]
                      frame False {
                        (unwired) FALSE ("y")
                        n133 = Unbundle By Name(w184) -> ("Main Screen.STOP"=w190:refnum<vi>)
                        n134 = Unbundle By Name(w184) -> ("Main Screen.Start Test"=w187:refnum<vi>)
                        n135 = Unbundle By Name(w184) -> ("Main Screen.Start Test Temp"=w198:refnum<vi>)
                        n136 = Unbundle By Name(w184) -> ("Main Screen.STOP"=w197:refnum<vi>)
                        n137 = property class="Bool (strict)"(reference=w190, "Visible"=FALSE) -> (reference out=w192:refnum<vi>, error out=w191:errorcluster)  [unwired: 1 in]
                        n138 = property class="Bool (strict)"(reference=w187, "Visible"=TRUE) -> (reference out=w185:refnum<vi>, error out=w186:errorcluster)  [unwired: 1 in]
                        n139 = property class="Bool (strict)"(reference=w198, "Value"=FALSE) -> (reference out=w200:refnum<vi>, error out=w199:errorcluster)  [unwired: 1 in]
                        n140 = property class="Bool (strict)"(reference=w197, "Value"=TRUE) -> (reference out=w195:refnum<vi>, error out=w196:errorcluster)  [unwired: 1 in]
                        n141 = Close Reference(reference=w192, error in (no error)=w191) -> ()  [unwired: 1 out]
                        n142 = Close Reference(reference=w185, error in (no error)=w186) -> ()  [unwired: 1 out]
                        n143 = Close Reference(reference=w200, error in (no error)=w199) -> ()  [unwired: 1 out]
                        n144 = Close Reference(reference=w195, error in (no error)=w196) -> ()  [unwired: 1 out]
                      }
                      frame True {
                      }
                    }
                  }
                  frame True {
                  }
                }
                "Test Stop Temp" <- TRUE ("Test Stop Temp")
              }
            }
            n145 = Close Reference(reference=w114, error in (no error)=w115) -> ()  [unwired: 1 out]
            n146 = Close Reference(reference=w105, error in (no error)=w106) -> ()  [unwired: 1 out]
            n147 = Unbundle By Name(w69) -> ("Main Screen.Cyclic Coefficient of Friction"=w98:refnum<vi>)
            n148 = Close Reference(reference=w90, error in (no error)=w91) -> ()  [unwired: 1 out]
            n149 = Unbundle By Name(w69) -> ("Main Screen.Coefficient of Friction"=w112:refnum<vi>)
            n150 = Divide(x=w101, y=w89) -> (x/y=w97:dbl)
            n151 = Divide(x=w110, y=w89) -> (x/y=w109:dbl)
            n152 = property class="WFChart (strict)"(reference=w112, "Value"=w109) -> (reference out=w113:refnum<vi>, error out=w111:errorcluster)  [unwired: 1 in]
            n153 = property class="WFChart (strict)"(reference=w98, "Value"=w97) -> (reference out=w96:refnum<vi>, error out=w99:errorcluster)  [unwired: 1 in]
            n154 = Close Reference(reference=w113, error in (no error)=w111) -> ()  [unwired: 1 out]
            n155 = Close Reference(reference=w96, error in (no error)=w99) -> ()  [unwired: 1 out]
          }
        }
      }
    }
    frame Error {
    }
  }
